vi "Math Finder.vi"(8 "error in (no error)":errorcluster, 11 "Get Tagged String":string) -> (0 "error out":errorcluster, 1 "in2":string, 2 "Expression":string, 3 "in1":string)   [LabVIEW 2014]
doc: "This VI takes tagged string from SBML parser.vi as input and translate it into kinetic law. It supports the following five mathematical functions:\n+, -, *, /, pow\n\nDesigned by HB\nhaba@dtu.dk"
uses:
  <vilib>/regexp/Match Regular Expression.xnode
panel:
  # "SOP3 pow SOP4 * SOP5 / kr_f kr_r EOP5 LacI EOP4 nc EOP3"
  # "SOP1 + x 2 EOP1"
  # "SOP1 + SOP2 * a b EOP2 c EOP1"
  # "SOP1 + c SOP2 * a b EOP2 EOP1"
  # "SOP1 + SOP2 * a SOP3 pow x 2 EOP3 EOP2 SOP2 * b x EOP2 c EOP1"
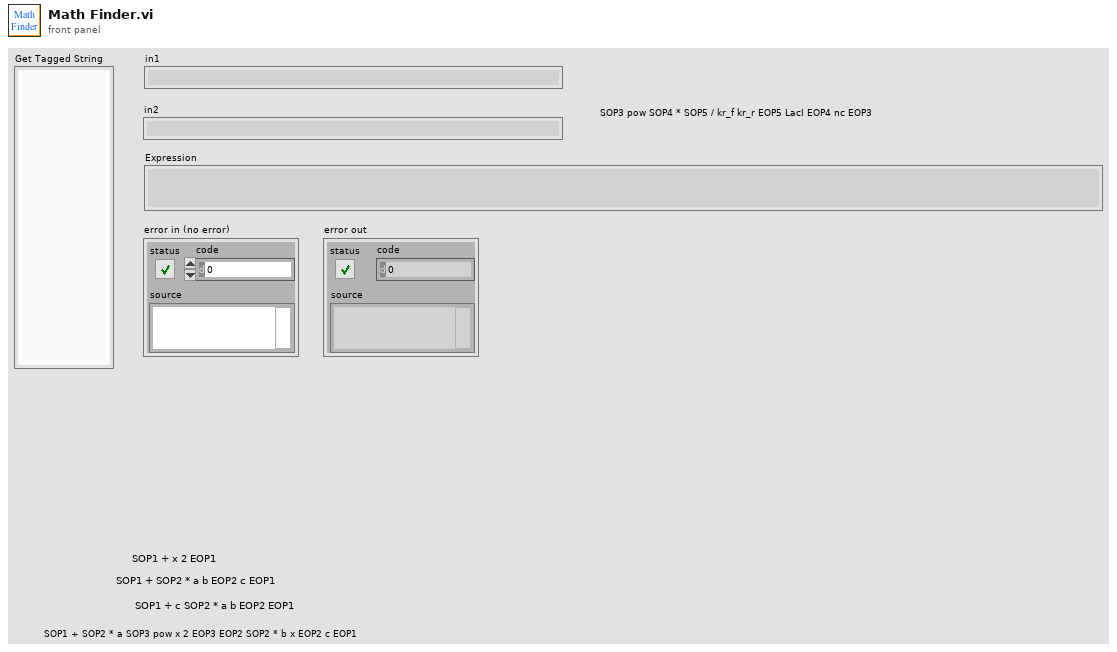
[diagram p1: front panel]
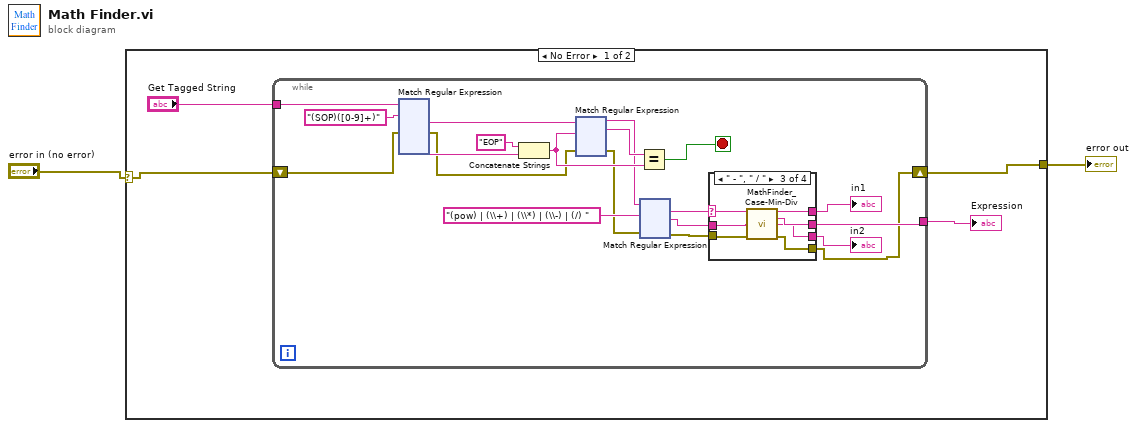
[diagram p0: block diagram]
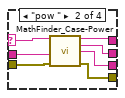
[diagram p3: hidden frame]
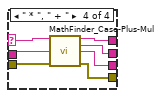
[diagram p4: hidden frame]
diagram:
  n1 = case shown="No Error" "error in (no error)" {
    selector: "error in (no error)" -> [w3 w394]
    tunnel: [w4 w394] -> w2
    frame No Error {
      n2 = while {
        tunnel: [w18] -> w5
        tunnel: "Get Tagged String" -> [w12]
        shift-right: [w7] -> w4
        shift-left: w3 -> [w11]
        stop <- w24 stop-if-true
        n3 = xnode "Match Regular Expression"("input string"=w12, "regular expression"="(SOP)([0-9]+)", "error in"=w11) -> ("after match"=w15:string, "error out"=w10:errorcluster, "submatch 2"=w14:string)  [unwired: 3 in, 4 out]
        n4 = Concatenate Strings("EOP" ("regular expression"), w14) -> (w25:string)
        n5 = xnode "Match Regular Expression"("input string"=w15, "regular expression"=w25, "error in"=w10) -> ("before match"=w21:string, "whole match"=w22:string, "error out"=w9:errorcluster)  [unwired: 3 in, 2 out]
        n6 = Equal?(x=w22, y=w25) -> (x = y?=w24:bool)
        n7 = xnode "Match Regular Expression"("input string"=w21, "regular expression"="(pow) | (\\+) | (\\*) | (\\-) | (/) " ("Oprts Lst"), "error in"=w9) -> ("whole match"=w23:string, "after match"=w20:string, "error out"=w8:errorcluster)  [unwired: 3 in, 2 out]
        n8 = case shown="\" - \", \" / \"" w23 {
          selector: w23 -> [_ w379 w386 w393]
          tunnel: w20 -> [_ w373 w382 w389]
          tunnel: [_ w377 w384 w391] -> w18
          tunnel: [_ w376 w383 w390] -> w17
          tunnel: [_ w378 w385 w392] -> w16
          tunnel: w8 -> [w372 w375 w381 w388]
          tunnel: [w372 w374 w380 w387] -> w7
          frame "False", Default {
          }
          frame "pow " {
            n9 = call "MathFinder_Case-Power.vi"("Whole Match"=w379, "After Match"=w373, "error in (no error)"=w375) -> ("in1"=w378:string, "Expression"=w377:string, "in2"=w376:string, "error out"=w374:errorcluster)  [unwired: 9 in]
          }
          frame " - ", " / " {
            n10 = call "MathFinder_Case-Min-Div.vi"("Whole Match"=w386, "After Match"=w382, "error in (no error)"=w381) -> ("in1"=w385:string, "Expression"=w384:string, "in2"=w383:string, "error out"=w380:errorcluster)  [unwired: 9 in]
          }
          frame " * ", " + " {
            n11 = call "MathFinder_Case-Plus-Mul.vi"("Whole Match"=w393, "After Match"=w389, "error in (no error)"=w388) -> ("in1"=w392:string, "Expression"=w391:string, "in2"=w390:string, "error out"=w387:errorcluster)  [unwired: 9 in]
          }
        }
        "in2" <- w17
        "in1" <- w16
      }
      "Expression" <- w5
    }
    frame Error {
    }
  }
  "error out" <- w2
